vi "Write Scrollbar Position.vi"(8 "error in (no error)":errorcluster, 10 "Position":u32, 11 "LargeScrollbar in":refnum<class "LargeScrollbar.lvclass">) -> (0 "error out":errorcluster, 3 "LargeScrollbar out":refnum<class "LargeScrollbar.lvclass">)   [LabVIEW 2015, in "LargeScrollbar.lvclass"]
uses:
  LargeScrollbar.lvclass
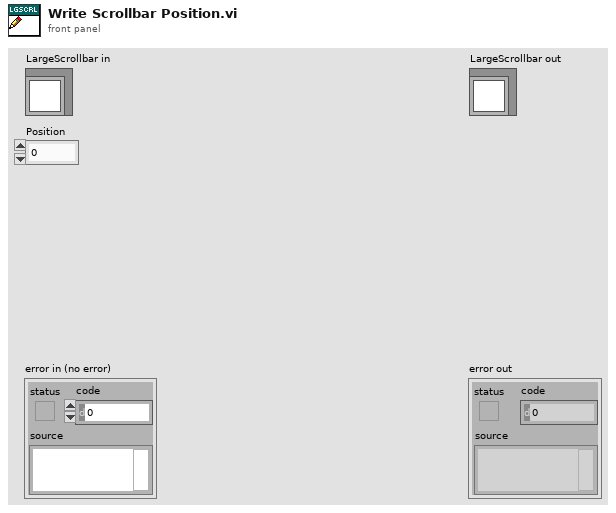
[diagram p1: front panel]
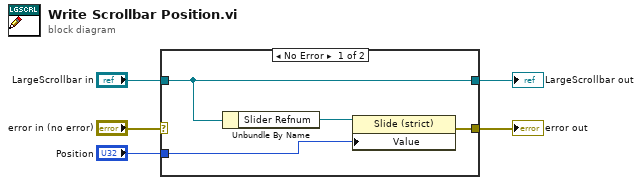
[diagram p0: block diagram]
diagram:
  n1 = case shown="No Error" "error in (no error)" {
    selector: "error in (no error)" -> [_ w11]
    tunnel: [w6 w11] -> w4
    tunnel: [w9 w10] -> w2
    tunnel: "LargeScrollbar in" -> [w9 w10]
    tunnel: "Position" -> [w7 _]
    frame No Error {
      n2 = Unbundle By Name(w9) -> ("Slider Refnum"=w8:refnum<vi>)
      n3 = property class="Slide (strict)"(reference=w8, "Value"=w7) -> (error out=w6:errorcluster)  [unwired: 1 in, 1 out]
    }
    frame Error {
    }
  }
  "error out" <- w4
  "LargeScrollbar out" <- w2
